vi "CfgRowHdr.vi"(9 "FundParamsRef":refnum<vi>, 10 "ParamsRef":refnum<vi>, 11 "PmuTestParams":dbl[][](array[numeric])) -> (4 "NormalType":bool)   [LabVIEW 2018, in "Functions.lvlib" / "PmuTestFunctions.lvclass"]
uses:
  PmuTestFunctions.lvclass
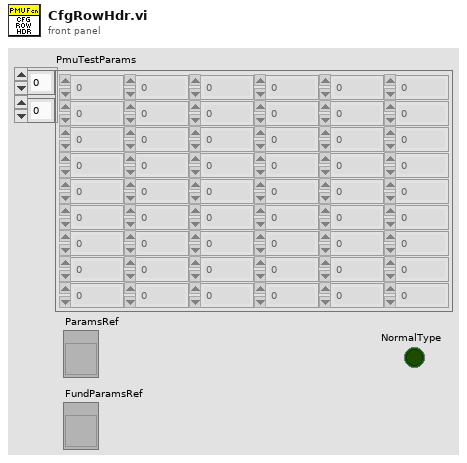
[diagram p1: front panel]
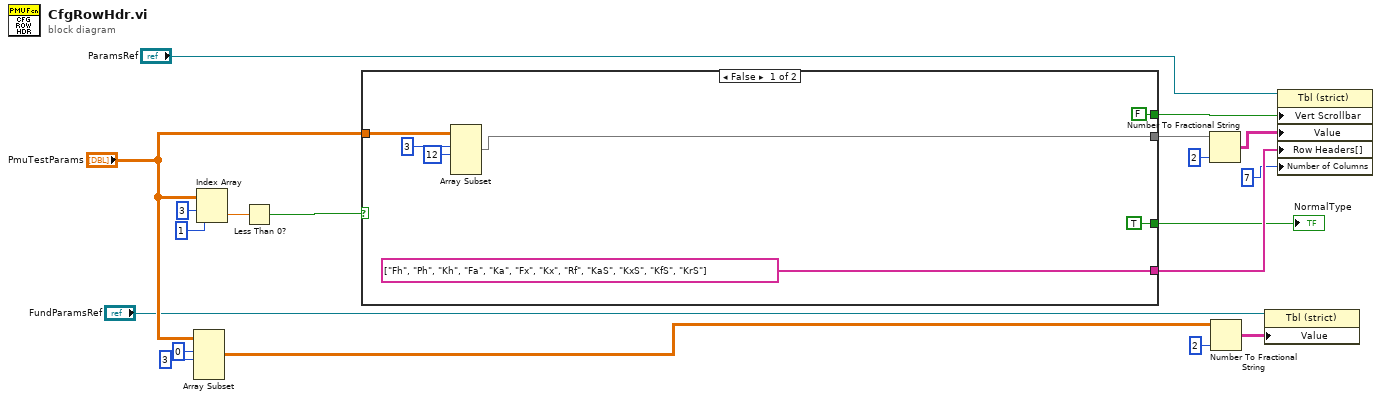
[diagram p0: block diagram]
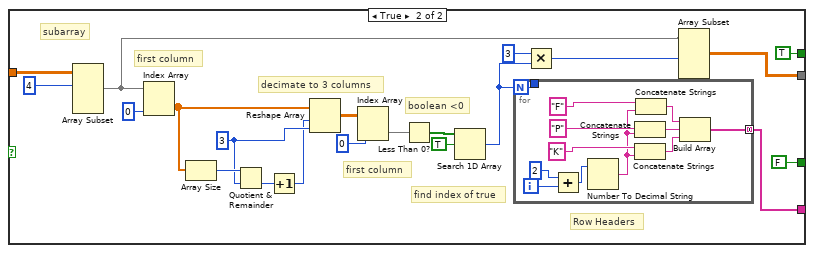
[diagram p2: hidden frame]
diagram:
  n1 = Array Subset(array="PmuTestParams", index (row)=0 ("index"), length (row)=3 ("length")) -> (w5:dbl[][])  [unwired: 2 in]
  n2 = Index Array(array="PmuTestParams", index (row)=3, index (col)=1 ("disabled index (col)")) -> (element=w17:dbl)
  n3 = Less Than 0?(x=w17) -> (x < 0?=w16:bool)
  n4 = case shown="False" w16 {
    tunnel: "PmuTestParams" -> [w26 w46]
    tunnel: [FALSE ("Visible Items:Vertical Scrollbar Visible") TRUE ("Visible Items:Vertical Scrollbar Visible")] -> w14
    tunnel: [string[] ["Fh", "Ph", "Kh", "Fa", "Ka", "Fx", "Kx", "Rf", "KaS", "KxS", "KfS", "KrS"] w33] -> w13
    tunnel: [w21 w28] -> w11
    tunnel: [TRUE FALSE] -> w1
    frame False {
      n5 = Array Subset(array=w26, index (row)=3 ("index"), length (row)=12 ("length")) -> (w21:dbl[][])  [unwired: 2 in]
    }
    frame True {
      w42 = 3 ("dimension size")
      # "Row Headers"
      # "find index of true"
      # "boolean <0"
      # "first column"
      # "decimate to 3 columns"
      # "first column"
      # "subarray"
      n6 = Array Subset(array=w46, index (row)=4 ("index")) -> (w30:dbl[][])  [unwired: 3 in]
      n7 = Index Array(array=w30, index (col)=0 ("disabled index (col)")) -> (element=w44:dbl[])  [unwired: 1 in]
      n8 = Array Size(array=w44) -> (size(s)=w43:i32)
      n9 = Quotient & Remainder(x=w43, y=w42) -> (floor(x/y)=w41:i32)  [unwired: 1 out]
      n10 = Increment(x=w41) -> (x+1=w40:i32)
      n11 = Reshape Array(w44, w40, w42) -> (w39:dbl[][])
      n12 = Index Array(array=w39, index (col)=0 ("disabled index (col)")) -> (element=w37:dbl[])  [unwired: 1 in]
      n13 = Less Than 0?(x=w37) -> (x < 0?=w36:bool[])
      n14 = Search 1D Array(1D array=w36, element=TRUE) -> (index of element=w32:i32)  [unwired: 1 in]
      n15 = for {
        N: w32 -> [w48]
        tunnel: [w49] -> w33 mode=concatenating
        tunnel: [w48] -> _
        i -> [w59]
        n16 = Add(x=2, y=w59) -> (x+y=w57:i32)
        n17 = Number To Decimal String(number=w57) -> (decimal integer string=w53:string)  [unwired: 1 in]
        n18 = Concatenate Strings("P", w53) -> (w51:string)
        n19 = Concatenate Strings("K", w53) -> (w50:string)
        n20 = Concatenate Strings("F", w53) -> (w52:string)
        n21 = Build Array(w52, w51, w50) -> (w49:string[])
      }
      n22 = Multiply(x=3, y=w32) -> (x*y=w29:i32)
      n23 = Array Subset(array=w30, length (row)=w29) -> (w28:dbl[][])  [unwired: 3 in]
    }
  }
  "NormalType" <- w1
  n24 = Number To Fractional String(number=w11, precision (6)=i16 2) -> (F-format string=w10:string[][])  [unwired: 2 in]
  n25 = Number To Fractional String(number=w5, precision (6)=i16 2) -> (F-format string=w3:string[][])  [unwired: 2 in]
  n26 = property class="Tbl (strict)"(reference="FundParamsRef", "Value"=w3) -> ()  [unwired: 1 in, 2 out]
  n27 = property class="Tbl (strict)"(reference="ParamsRef", "Vert Scrollbar"=w14, "Value"=w10, "Row Headers[]"=w13, "Number of Columns"=u32 7) -> ()  [unwired: 1 in, 2 out]
